vi "灯组解析.vi"() -> ()   [LabVIEW 2015]
uses:
  <userlib>/QMH/Message Queue/Support/Enqueue Message (Single).vi
  Global control/global-1.vi
  <vilib>/Instr/_visa.llb/VISA Configure Serial Port (Instr).vi
  <userlib>/QMH/Message Queue/Support/Enqueue Message (Array).vi
  <userlib>/QMH/Message Queue/Message Queue.lvlib
  <userlib>/QMH/User Event - Stop/User Event - Stop.lvlib
panel:
  in  "HostThread":variant
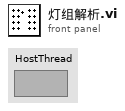
[diagram p1: front panel]
types:
  T1 = cluster{"Controls":cluster{"Exit":refnum<vi>}, "Thread":cluster{"ThisQ":string, "ThisVI":refnum<vi>, "HostQ":string, "HostRef":refnum<vi>, "SlavesQ":string[], "SlavesRef":refnum<vi>[]}, "Data":cluster{"Replace":bool}, "User":cluster{"Name":string}, "长度1-1":cluster{"225":bool, "201":bool, "202":bool, "226":bool, "236":bool, "236-7":bool, "237":bool, "237-7":bool, "231":bool, "231-7":bool, "245":bool, "2451":bool, "241":bool, "241-7":bool, "备用1":bool, "备用2":bool}, "长度2":cluster{"65":bool, "75":bool, "401":bool, "402":bool, "445":bool, "404":bool, "213":bool, "2130":bool, "2131":bool, "405":bool, "406":bool, "407":bool, "备用1":bool, "备用2":bool, "备用3":bool, "备用4":bool}, "长度1-2":cluster{"60":bool, "70":bool, "2120":bool, "212":bool, "2121":bool, "2124":bool, "214":bool, "2140":bool, "2141":bool, "90":bool, "2110":bool, "211":bool, "2111":bool, "2113":bool, "备用1":bool, "备用2":bool}, "VISA":refnum<visa-resource-name>, "1-1":cluster{"225":refnum<vi>, "201":refnum<vi>, "202":refnum<vi>, "226":refnum<vi>, "236":refnum<vi>, "236-7":refnum<vi>, "237":refnum<vi>, "237-7":refnum<vi>, "231":refnum<vi>, "231-7":refnum<vi>, "245":refnum<vi>, "2451":refnum<vi>, "241":refnum<vi>, "241-7":refnum<vi>}, "1-2":cluster{"60":refnum<vi>, "70":refnum<vi>, "2120":refnum<vi>, "212":refnum<vi>, "2121":refnum<vi>, "2124":refnum<vi>, "214":refnum<vi>, "2140":refnum<vi>, "2141":refnum<vi>, "90":refnum<vi>, "2110":refnum<vi>, "211":refnum<vi>, "2111":refnum<vi>, "2113":refnum<vi>}, "2":cluster{"65":refnum<vi>, "75":refnum<vi>, "401":refnum<vi>, "402":refnum<vi>, "445":refnum<vi>, "404":refnum<vi>, "213":refnum<vi>, "2130":refnum<vi>, "2131":refnum<vi>, "405":refnum<vi>, "406":refnum<vi>, "407":refnum<vi>}}
  T2 = cluster{"1-1":cluster{"225":refnum<vi>, "201":refnum<vi>, "202":refnum<vi>, "226":refnum<vi>, "236":refnum<vi>, "236-7":refnum<vi>, "237":refnum<vi>, "237-7":refnum<vi>, "231":refnum<vi>, "231-7":refnum<vi>, "245":refnum<vi>, "2451":refnum<vi>, "241":refnum<vi>, "241-7":refnum<vi>}, "1-2":cluster{"60":refnum<vi>, "70":refnum<vi>, "2120":refnum<vi>, "212":refnum<vi>, "2121":refnum<vi>, "2124":refnum<vi>, "214":refnum<vi>, "2140":refnum<vi>, "2141":refnum<vi>, "90":refnum<vi>, "2110":refnum<vi>, "211":refnum<vi>, "2111":refnum<vi>, "2113":refnum<vi>}, "2":cluster{"65":refnum<vi>, "75":refnum<vi>, "401":refnum<vi>, "402":refnum<vi>, "445":refnum<vi>, "404":refnum<vi>, "213":refnum<vi>, "2130":refnum<vi>, "2131":refnum<vi>, "405":refnum<vi>, "406":refnum<vi>, "407":refnum<vi>}}
  T3 = cluster{"225":bool, "201":bool, "202":bool, "226":bool, "236":bool, "236-7":bool, "237":bool, "237-7":bool, "231":bool, "231-7":bool, "245":bool, "2451":bool, "241":bool, "241-7":bool, "备用1":bool, "备用2":bool}
  T4 = cluster{"225":refnum<vi>, "201":refnum<vi>, "202":refnum<vi>, "226":refnum<vi>, "236":refnum<vi>, "236-7":refnum<vi>, "237":refnum<vi>, "237-7":refnum<vi>, "231":refnum<vi>, "231-7":refnum<vi>, "245":refnum<vi>, "2451":refnum<vi>, "241":refnum<vi>, "241-7":refnum<vi>}
  T5 = cluster{"60":refnum<vi>, "70":refnum<vi>, "2120":refnum<vi>, "212":refnum<vi>, "2121":refnum<vi>, "2124":refnum<vi>, "214":refnum<vi>, "2140":refnum<vi>, "2141":refnum<vi>, "90":refnum<vi>, "2110":refnum<vi>, "211":refnum<vi>, "2111":refnum<vi>, "2113":refnum<vi>}
  T6 = cluster{"65":refnum<vi>, "75":refnum<vi>, "401":refnum<vi>, "402":refnum<vi>, "445":refnum<vi>, "404":refnum<vi>, "213":refnum<vi>, "2130":refnum<vi>, "2131":refnum<vi>, "405":refnum<vi>, "406":refnum<vi>, "407":refnum<vi>}
  T7 = cluster{"60":bool, "70":bool, "2120":bool, "212":bool, "2121":bool, "2124":bool, "214":bool, "2140":bool, "2141":bool, "90":bool, "2110":bool, "211":bool, "2111":bool, "2113":bool, "备用1":bool, "备用2":bool}
  T8 = cluster{"65":bool, "75":bool, "401":bool, "402":bool, "445":bool, "404":bool, "213":bool, "2130":bool, "2131":bool, "405":bool, "406":bool, "407":bool, "备用1":bool, "备用2":bool, "备用3":bool, "备用4":bool}
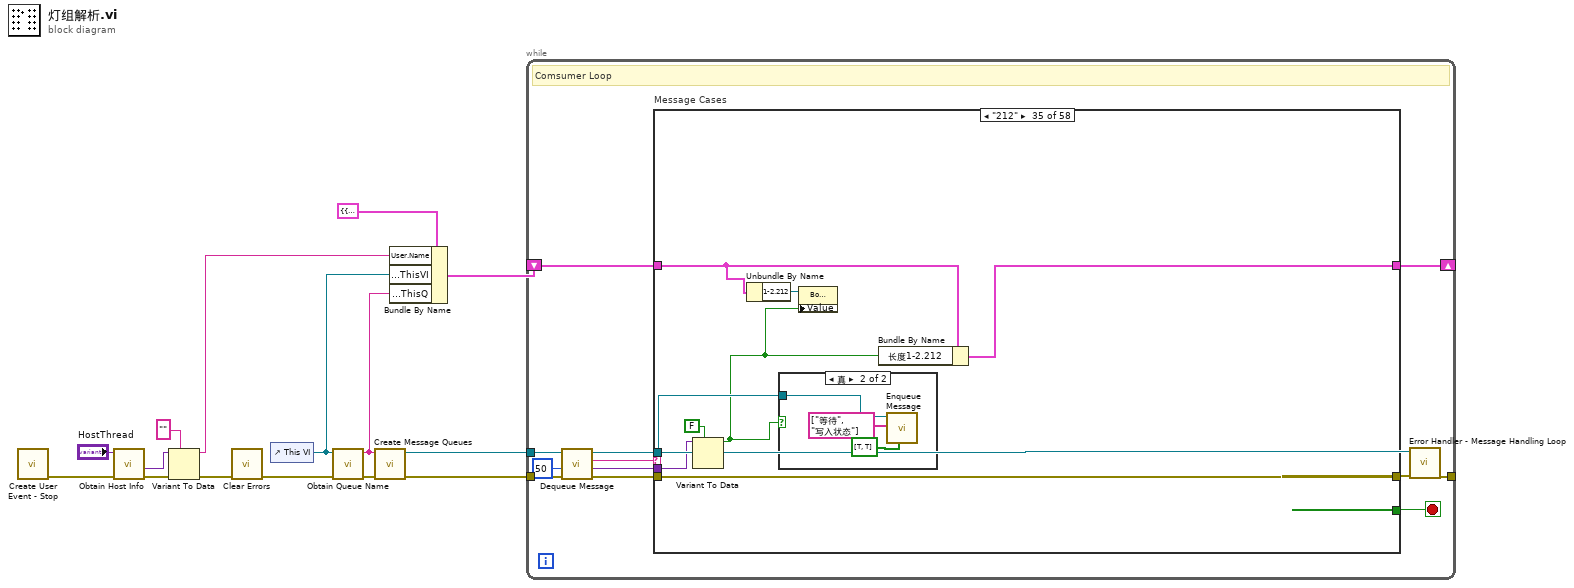
[diagram p0: block diagram]
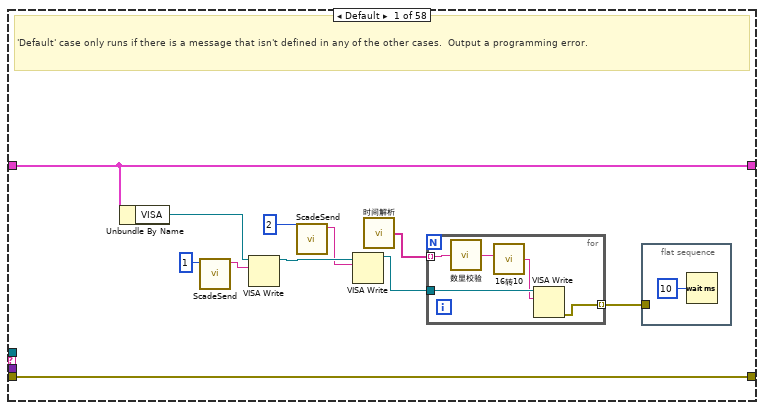
[diagram p2: hidden frame]
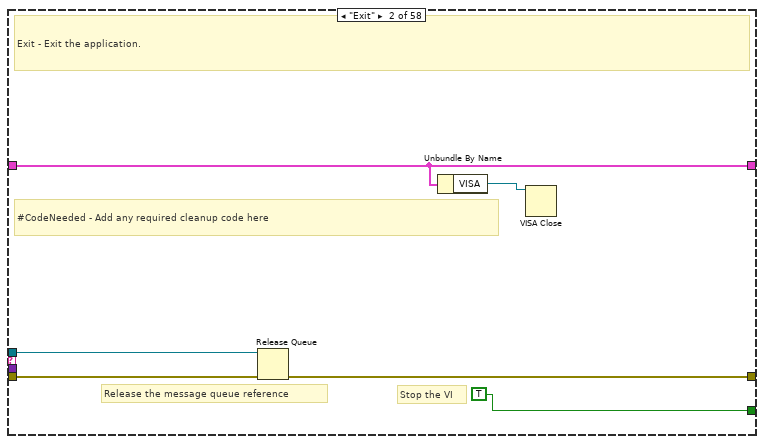
[diagram p3: hidden frame]
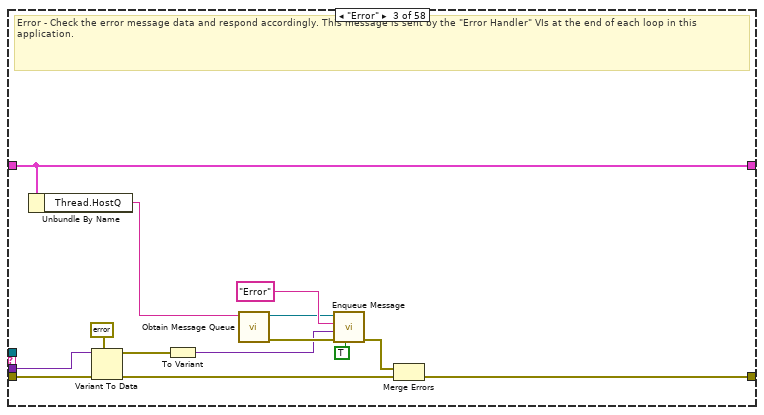
[diagram p4: hidden frame]
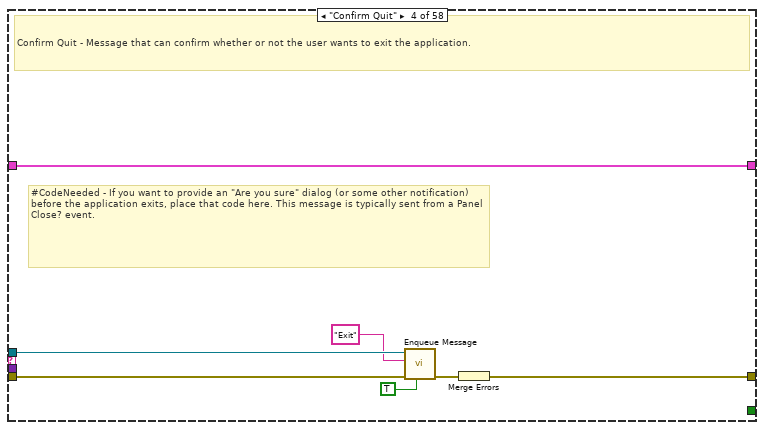
[diagram p5: hidden frame]
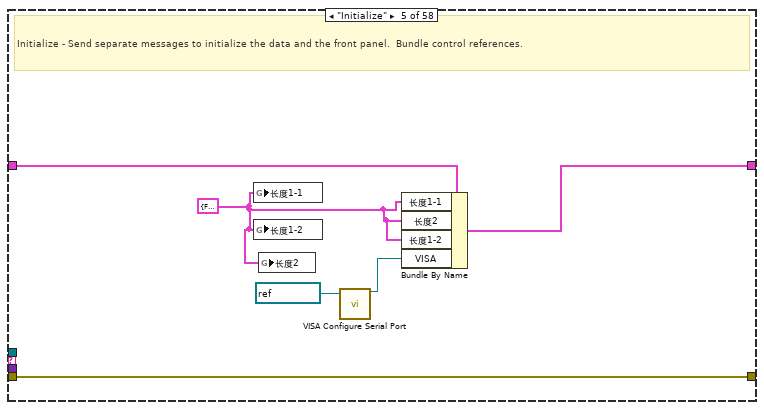
[diagram p6: hidden frame]
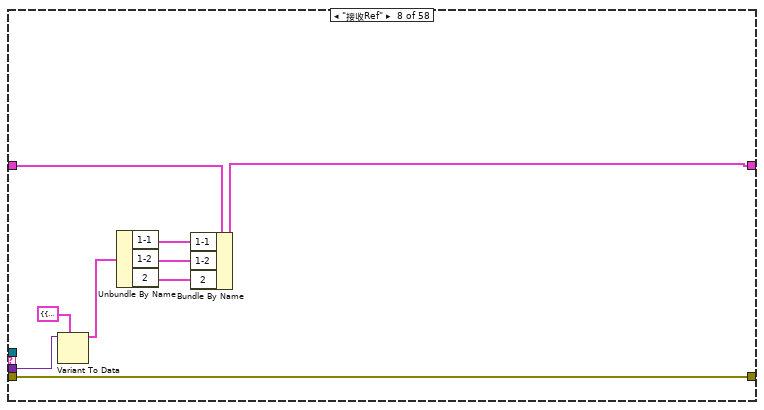
[diagram p9: hidden frame]
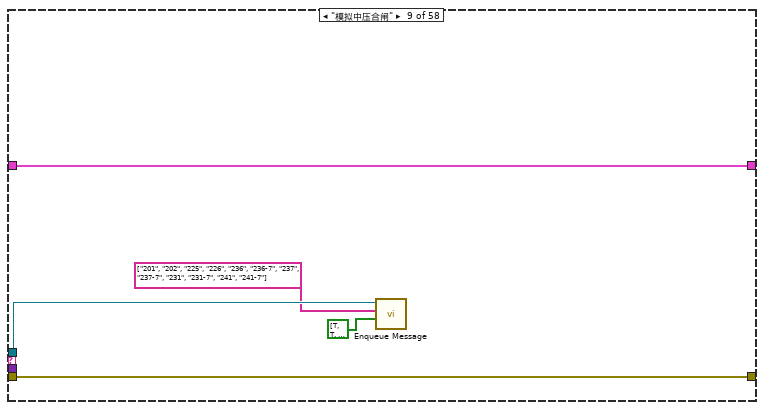
[diagram p10: hidden frame]
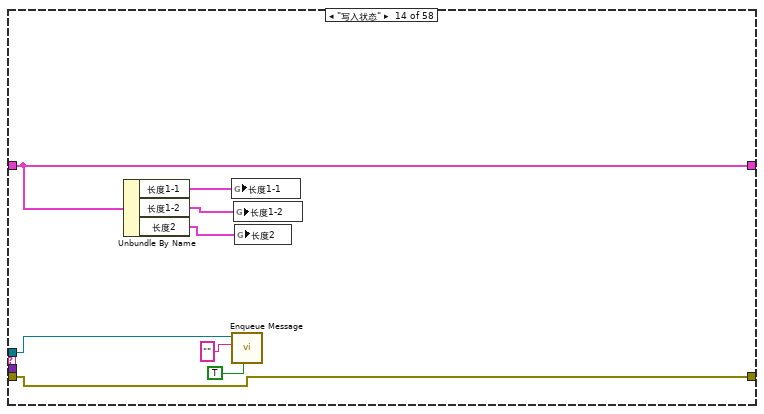
[diagram p15: hidden frame]
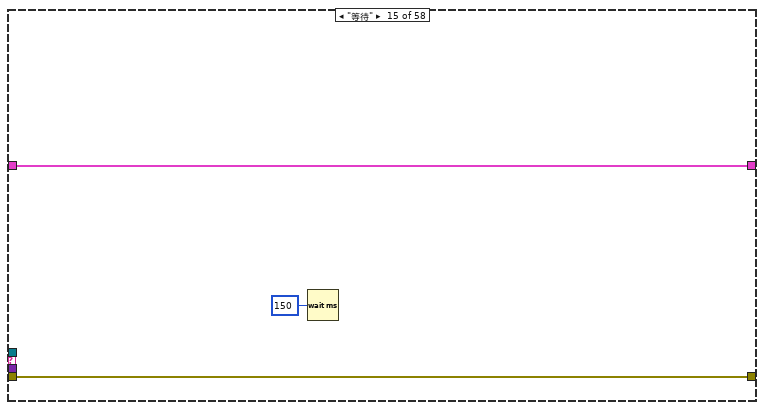
[diagram p16: hidden frame]
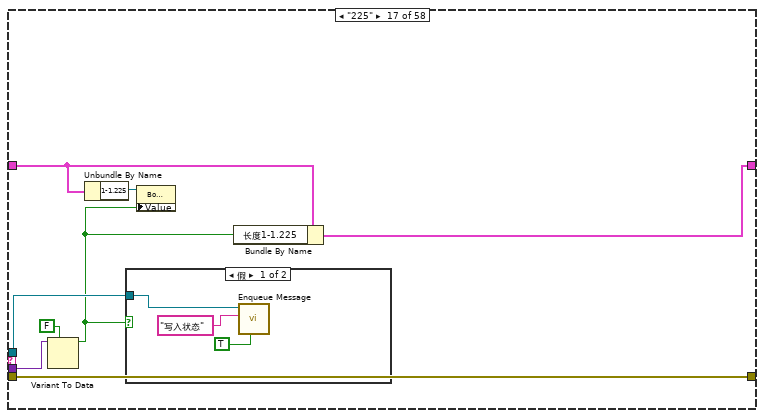
[diagram p18: hidden frame]
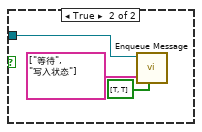
[diagram p19: hidden frame]
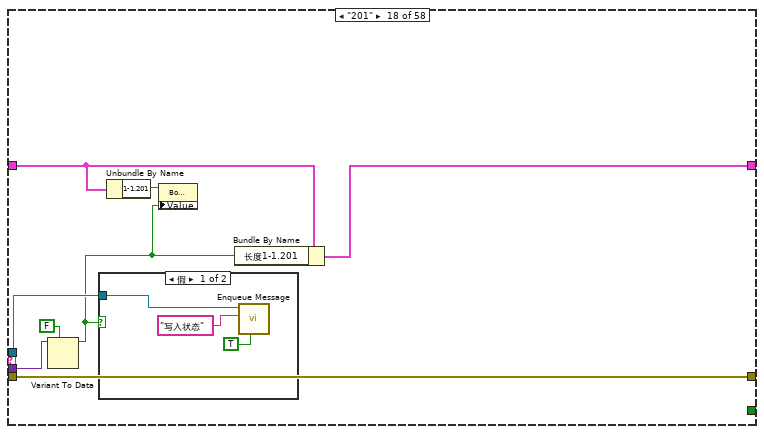
[diagram p20: hidden frame]
diagram:
  n1 = call <userlib>:"Create User Event - Stop.vi"() -> ("error out"=w9:errorcluster)  [unwired: 9 in, 2 out]
  n2 = call <userlib>:"Obtain Host Info.vi"("error in (no error)"=w9, "HostThread"="HostThread") -> ("error out"=w7:errorcluster, "Data"=w6:variant)  [unwired: 6 in, 2 out]
  n3 = Variant To Data(error in=w7, type="", Variant=w6) -> (data=w2:string, error out=w4:errorcluster)
  n4 = call <vilib>:"Clear Errors.vi"("error in (no error)"=w4) -> ("error out"=w3:errorcluster)  [unwired: 5 in, 1 out]
  n5 = control-ref of="This VI"() -> (w11:refnum<vi>)
  n6 = call <userlib>:"Obtain Queue Name.vi"("error in (no error)"=w3, "VI Refnum"=w11) -> ("error out"=w14:errorcluster, "ViName"=w10:string)  [unwired: 8 in]
  n7 = call <userlib>:"Create Message Queues.vi"("error in (no error)"=w14, "name (unnamed)"=w10) -> ("error out"=w15:errorcluster, "QueueHandler"=w1:refnum<queue>)  [unwired: 8 in]
  n8 = Bundle By Name(cluster=T1 {"Controls"={"Exit"=refnum}, "Thread"={"ThisQ"="", "ThisVI"=refnum, "HostQ"="", "HostRef"=refnum, "SlavesQ"=[], "SlavesRef"=[]}, "Data"={"Replace"=FALSE}, "User"={"Name"=""}, "长度1-1"={"225"=FALSE, "201"=FALSE, "202"=FALSE, "226"=FALSE, "236"=FALSE, "236-7"=FALSE, "237"=FALSE, "237-7"=FALSE, "231"=FALSE, "231-7"=FALSE, "245"=FALSE, "2451"=FALSE, "241"=FALSE, "241-7"=FALSE, "备用1"=FALSE, "备用2"=FALSE}, "长度2"={"65"=FALSE, "75"=FALSE, "401"=FALSE, "402"=FALSE, "445"=FALSE, "404"=FALSE, "213"=FALSE, "2130"=FALSE, "2131"=FALSE, "405"=FALSE, "406"=FALSE, "407"=FALSE, "备用1"=FALSE, "备用2"=FALSE, "备用3"=FALSE, "备用4"=FALSE}, "长度1-2"={"60"=FALSE, "70"=FALSE, "2120"=FALSE, "212"=FALSE, "2121"=FALSE, "2124"=FALSE, "214"=FALSE, "2140"=FALSE, "2141"=FALSE, "90"=FALSE, "2110"=FALSE, "211"=FALSE, "2111"=FALSE, "2113"=FALSE, "备用1"=FALSE, "备用2"=FALSE}, "VISA"="", "1-1"={"225"=refnum, "201"=refnum, "202"=refnum, "226"=refnum, "236"=refnum, "236-7"=refnum, "237"=refnum, "237-7"=refnum, "231"=refnum, "231-7"=refnum, "245"=refnum, "2451"=refnum, "241"=refnum, "241-7"=refnum}, "1-2"={"60"=refnum, "70"=refnum, "2120"=refnum, "212"=refnum, "2121"=refnum, "2124"=refnum, "214"=refnum, "2140"=refnum, "2141"=refnum, "90"=refnum, "2110"=refnum, "211"=refnum, "2111"=refnum, "2113"=refnum}, "2"={"65"=refnum, "75"=refnum, "401"=refnum, "402"=refnum, "445"=refnum, "404"=refnum, "213"=refnum, "2130"=refnum, "2131"=refnum, "405"=refnum, "406"=refnum, "407"=refnum}} ("Data Cluster"), "User.Name"=w2, "Thread.ThisVI"=w11, "Thread.ThisQ"=w10) -> (w12:T1)
  n9 = while {
    tunnel: w1 -> [w20]
    shift-right: [w26] -> _
    shift-left: w12 -> [w27]
    tunnel: w15 -> [w24]
    tunnel: [w18] -> _
    stop <- w25 stop-if-true
    # "Comsumer Loop"
    n10 = call <userlib>:"Dequeue Message.vi"("error in (no error)"=w24, "timeout in ms (-1)"=50, "Message Queue"=w20) -> ("error out"=w23:errorcluster, "Message Data"=w21:variant, "Message"=w22:string, "dup Message Queue"=w19:refnum<queue>)  [unwired: 5 in]
    n11 = case "Message Cases" shown="\"212\"" w22 {
      tunnel: w19 -> [_ w50 _ w67 _ _ _ _ w93 _ _ _ _ w106 _ _ w120 w134 w148 w162 w176 w190 w204 w218 w232 w246 w260 w274 w288 w302 _ w318 w332 w346 w360 w374 w388 w402 w416 w430 w444 w458 w472 w486 w500 _ w516 w530 w544 w558 w572 w586 w600 w614 w628 w642 w656 w670]
      tunnel: w23 -> [w30 w48 w64 w71 w77 w79 w81 w90 w95 w97 w98 w101 w103 w111 w114 w116 w124 w138 w152 w166 w180 w194 w208 w222 w236 w250 w264 w278 w292 w306 w314 w322 w336 w350 w364 w378 w392 w406 w420 w434 w448 w462 w476 w490 w504 w512 w520 w534 w548 w562 w576 w590 w604 w618 w632 w646 w660 w674]
      tunnel: [w30 w47 w59 w69 w77 w79 w81 w90 w95 w97 w98 w101 w103 w111 w114 w116 w124 w138 w152 w166 w180 w194 w208 w222 w236 w250 w264 w278 w292 w306 w314 w322 w336 w350 w364 w378 w392 w406 w420 w434 w448 w462 w476 w490 w504 w512 w520 w534 w548 w562 w576 w590 w604 w618 w632 w646 w660 w674] -> w17
      tunnel: w27 -> [w32 w46 w56 w70 w74 w78 w80 w83 w94 w96 w99 w100 w102 w110 w113 w115 w119 w132 w147 w160 w174 w188 w202 w216 w230 w244 w258 w272 w286 w300 w313 w316 w330 w344 w358 w372 w386 w400 w414 w428 w442 w456 w470 w484 w498 w511 w514 w528 w542 w556 w570 w584 w598 w612 w626 w640 w654 w668]
      tunnel: [w32 w46 w56 w70 w73 w78 w80 w82 w94 w96 w99 w100 w102 w110 w113 w115 w121 w135 w149 w163 w177 w191 w205 w219 w233 w247 w261 w275 w289 w303 w313 w319 w333 w347 w361 w375 w389 w403 w417 w431 w445 w459 w473 w487 w501 w511 w517 w531 w545 w559 w573 w587 w601 w615 w629 w643 w657 w671] -> w26
      tunnel: [_ TRUE _ _ _ _ _ _ _ _ _ _ _ _ _ _ _ _ _ _ _ _ _ _ _ _ _ _ _ _ _ _ _ _ _ _ _ _ _ _ _ _ _ _ _ _ _ _ _ _ _ _ _ _ _ _ _ _] -> w25
      tunnel: w21 -> [_ _ w63 _ _ _ _ w89 _ _ _ _ _ _ _ _ w123 w137 w151 w165 w179 w193 w207 w221 w235 w249 w263 w277 w291 w305 _ w321 w335 w349 w363 w377 w391 w405 w419 w433 w447 w461 w475 w489 w503 _ w519 w533 w547 w561 w575 w589 w603 w617 w631 w645 w659 w673]
      frame Default {
        # "'Default' case only runs if there is a message that isn't defined in any of the other cases.  Output a programming error."
        n12 = Unbundle By Name(w32) -> ("VISA"=w31:refnum<visa-resource-name>)
        n13 = call "ScadeSend.vi"("长度"=1) -> ("String"=w36:string)  [unwired: 10 in]
        n14 = VISA Write(VISA resource name=w31, write buffer=w36) -> (VISA resource name out=w35:refnum<visa-resource-name>)  [unwired: 1 in, 2 out]
        n15 = call "ScadeSend.vi"("长度"=2 ("长度 2")) -> ("String"=w34:string)  [unwired: 10 in]
        n16 = VISA Write(VISA resource name=w35, write buffer=w34) -> (VISA resource name out=w37:refnum<visa-resource-name>)  [unwired: 1 in, 2 out]
        n17 = call "时间解析.vi"() -> ("数组"=w33:string[])
        n18 = for {
          tunnel: w33 -> [w41] mode=indexing
          tunnel: w37 -> [w43]
          tunnel: [w40] -> w28 mode=indexing
          n19 = call "数显校验.vi"("字符串"=w41) -> ("连接的字符串"=w44:string)
          n20 = call "16转10.vi"("字符串"=w44) -> ("字符串 2"=w42:string)
          n21 = VISA Write(VISA resource name=w43, write buffer=w42) -> (error out=w40:errorcluster)  [unwired: 1 in, 2 out]
        }
        n22 = flat-sequence {
          tunnel: w28 -> [_]
          frame #0 {
            n23 = Wait (ms)(milliseconds to wait=u32 10 ("等待时间（毫秒）")) -> ()  [unwired: 1 out]
          }
        }
      }
      frame "Exit" {
        # "Stop the VI"
        # "Release the message queue reference"
        # "#CodeNeeded - Add any required cleanup code here"
        # "Exit - Exit the application."
        n24 = Release Queue(queue=w50, error in (no error)=w48) -> (error out=w47:errorcluster)  [unwired: 1 in, 2 out]
        n25 = Unbundle By Name(w46) -> ("VISA"=w45:refnum<visa-resource-name>)
        n26 = VISA Close(VISA resource name=w45) -> ()  [unwired: 1 in, 1 out]
      }
      frame "Error" {
        # "Error - Check the error message data and respond accordingly. This message is sent by the \"Error Handler\" VIs at the end of each loop in this application."
        n27 = Unbundle By Name(w56) -> ("Thread.HostQ"=w55:string)
        n28 = Variant To Data(error in=w64, type=errorcluster {"status"=FALSE, "code"=0, "source"=""} ("error constant"), Variant=w63) -> (data=w52:errorcluster, error out=w61:errorcluster)
        n29 = To Variant(anything=w52) -> (Variant=w51:variant)
        n30 = call <userlib>:"Obtain Message Queue.vi"("name (unnamed)"=w55) -> ("error out"=w54:errorcluster, "Message Queue"=w53:refnum<queue>)  [unwired: 9 in]
        n31 = call-poly <userlib>:"Enqueue Message.vi"("Priority Message? (F)"=TRUE, "error in (no error)"=w54, "Message Data"=w51, "Message"="Error", "Message Queue"=w53) -> ("error out"=w60:errorcluster)  [unwired: 5 in, 1 out]
        n32 = Merge Errors(w60, w61) -> (w59:errorcluster)
      }
      frame "Confirm Quit" {
        # "#CodeNeeded - If you want to provide an \"Are you sure\" dialog (or some other notification) before the application exits, place that code here. This message is typically sent from a Panel Close? event."
        # "Confirm Quit - Message that can confirm whether or not the user wants to exit the application."
        n33 = call-poly <userlib>:"Enqueue Message.vi"("Priority Message? (F)"=TRUE, "error in (no error)"=w71, "Message"="Exit", "Message Queue"=w67) -> ("error out"=w68:errorcluster)  [unwired: 6 in, 1 out]
        n34 = Merge Errors(w68) -> (w69:errorcluster)
      }
      frame "Initialize" {
        w76 = T3 {"225"=FALSE, "201"=FALSE, "202"=FALSE, "226"=FALSE, "236"=FALSE, "236-7"=FALSE, "237"=FALSE, "237-7"=FALSE, "231"=FALSE, "231-7"=FALSE, "245"=FALSE, "2451"=FALSE, "241"=FALSE, "241-7"=FALSE, "备用1"=FALSE, "备用2"=FALSE} ("长度1-1")
        # "Initialize - Send separate messages to initialize the data and the front panel.  Bundle control references."
        n35 = global write "global-1.vi" "长度1-1"(w76) -> ()
        n36 = global write "global-1.vi" "长度1-2"(w76) -> ()
        n37 = global write "global-1.vi" "长度2"(w76) -> ()
        n38 = call-poly "VISA Configure Serial Port"("VISA resource name"=refnum<visa-resource-name> "COM7" ("VISA资源名称")) -> ("VISA resource name out"=w72:refnum<visa-resource-name>)  [unwired: 8 in, 6 out]
        n39 = Bundle By Name(cluster=w74, "长度1-1"=w76, "长度2"=w76, "长度1-2"=w76, "VISA"=w72) -> (w73:T1)
      }
      frame "<-------UI-------->" {
      }
      frame "<------Core------>" {
      }
      frame "接收Ref" {
        n40 = Variant To Data(type=T2 {"1-1"={"225"=refnum, "201"=refnum, "202"=refnum, "226"=refnum, "236"=refnum, "236-7"=refnum, "237"=refnum, "237-7"=refnum, "231"=refnum, "231-7"=refnum, "245"=refnum, "2451"=refnum, "241"=refnum, "241-7"=refnum}, "1-2"={"60"=refnum, "70"=refnum, "2120"=refnum, "212"=refnum, "2121"=refnum, "2124"=refnum, "214"=refnum, "2140"=refnum, "2141"=refnum, "90"=refnum, "2110"=refnum, "211"=refnum, "2111"=refnum, "2113"=refnum}, "2"={"65"=refnum, "75"=refnum, "401"=refnum, "402"=refnum, "445"=refnum, "404"=refnum, "213"=refnum, "2130"=refnum, "2131"=refnum, "405"=refnum, "406"=refnum, "407"=refnum}} ("输出簇"), Variant=w89) -> (data=w87:T2)  [unwired: 1 in, 1 out]
        n41 = Unbundle By Name(w87) -> ("1-1"=w86:T4, "1-2"=w85:T5, "2"=w84:T6)
        n42 = Bundle By Name(cluster=w83, "1-1"=w86, "1-2"=w85, "2"=w84) -> (w82:T1)
      }
      frame "模拟中压合闸" {
        n43 = call-poly <userlib>:"Enqueue Message.vi"("Message Data Array"=bool[] [TRUE, TRUE, TRUE, TRUE, TRUE, TRUE, TRUE, TRUE, TRUE, TRUE, TRUE, TRUE], "Message Array"=string[] ["201", "202", "225", "226", "236", "236-7", "237", "237-7", "231", "231-7", "241", "241-7"], "Message Queue"=w93) -> ()  [unwired: 7 in, 2 out]
      }
      frame "顺序点亮" {
      }
      frame "Core_InitializeRef" {
        # "Initialize control references. For there is not enough space to locate all the control references, separate the codes into 2 messages"
      }
      frame "send" {
      }
      frame "<---Operation--->" {
      }
      frame "写入状态" {
        n44 = Unbundle By Name(w110) -> ("长度1-1"=w109:T3, "长度1-2"=w108:T7, "长度2"=w107:T8)
        n45 = global write "global-1.vi" "长度1-1"(w109) -> ()
        n46 = call-poly <userlib>:"Enqueue Message.vi"("Priority Message? (F)"=TRUE, "Message"="", "Message Queue"=w106) -> ()  [unwired: 7 in, 2 out]
        n47 = global write "global-1.vi" "长度1-2"(w108) -> ()
        n48 = global write "global-1.vi" "长度2"(w107) -> ()
      }
      frame "等待" {
        n49 = Wait (ms)(milliseconds to wait=u32 150 ("等待时间（毫秒）")) -> ()  [unwired: 1 out]
      }
      frame "<-------1-1------->" {
      }
      frame "225" {
        n50 = Variant To Data(type=FALSE, Variant=w123) -> (data=w117:bool)  [unwired: 1 in, 1 out]
        n51 = Unbundle By Name(w119) -> ("1-1.225"=w118:refnum<vi>)
        n52 = case shown="假" w117 {
          tunnel: w120 -> [w127 w130]
          frame False {
            n53 = call-poly <userlib>:"Enqueue Message.vi"("Priority Message? (F)"=TRUE, "Message"="写入状态", "Message Queue"=w127) -> ()  [unwired: 7 in, 2 out]
          }
          frame True {
            n54 = call-poly <userlib>:"Enqueue Message.vi"("Priority Message? Array"=bool[] [TRUE, TRUE], "Message Array"=string[] ["等待", "写入状态"] ("Message"), "Message Queue"=w130) -> ()  [unwired: 7 in, 2 out]
          }
        }
        n55 = property class="Bool (严格)"(reference=w118, "Value"=w117) -> ()  [unwired: 1 in, 2 out]
        n56 = Bundle By Name(cluster=w119, "长度1-1.225"=w117) -> (w121:T1)
      }
      frame "201" {
        n57 = Variant To Data(type=FALSE, Variant=w137) -> (data=w131:bool)  [unwired: 1 in, 1 out]
        n58 = case shown="假" w131 {
          tunnel: w134 -> [w141 w144]
          frame False {
            n59 = call-poly <userlib>:"Enqueue Message.vi"("Priority Message? (F)"=TRUE, "Message"="写入状态", "Message Queue"=w141) -> ()  [unwired: 7 in, 2 out]
          }
          frame True {
            n60 = call-poly <userlib>:"Enqueue Message.vi"("Priority Message? Array"=bool[] [TRUE, TRUE], "Message Array"=string[] ["等待", "写入状态"] ("Message"), "Message Queue"=w144) -> ()  [unwired: 7 in, 2 out]
          }
        }
        n61 = Unbundle By Name(w132) -> ("1-1.201"=w133:refnum<vi>)
        n62 = property class="Bool (严格)"(reference=w133, "Value"=w131) -> ()  [unwired: 1 in, 2 out]
        n63 = Bundle By Name(cluster=w132, "长度1-1.201"=w131) -> (w135:T1)
      }
      frame "202" {
        n64 = Variant To Data(type=FALSE, Variant=w151) -> (data=w145:bool)  [unwired: 1 in, 1 out]
        n65 = Unbundle By Name(w147) -> ("1-1.202"=w146:refnum<vi>)
        n66 = case shown="真" w145 {
          tunnel: w148 -> [w155 w158]
          frame False {
            n67 = call-poly <userlib>:"Enqueue Message.vi"("Priority Message? (F)"=TRUE, "Message"="写入状态", "Message Queue"=w155) -> ()  [unwired: 7 in, 2 out]
          }
          frame True {
            n68 = call-poly <userlib>:"Enqueue Message.vi"("Priority Message? Array"=bool[] [TRUE, TRUE], "Message Array"=string[] ["等待", "写入状态"] ("Message"), "Message Queue"=w158) -> ()  [unwired: 7 in, 2 out]
          }
        }
        n69 = property class="Bool (严格)"(reference=w146, "Value"=w145) -> ()  [unwired: 1 in, 2 out]
        n70 = Bundle By Name(cluster=w147, "长度1-1.202"=w145) -> (w149:T1)
      }
      frame "226" {
        n71 = Variant To Data(type=FALSE, Variant=w165) -> (data=w159:bool)  [unwired: 1 in, 1 out]
        n72 = Unbundle By Name(w160) -> ("1-1.226"=w161:refnum<vi>)
        n73 = case shown="真" w159 {
          tunnel: w162 -> [w169 w172]
          frame False {
            n74 = call-poly <userlib>:"Enqueue Message.vi"("Priority Message? (F)"=TRUE, "Message"="写入状态", "Message Queue"=w169) -> ()  [unwired: 7 in, 2 out]
          }
          frame True {
            n75 = call-poly <userlib>:"Enqueue Message.vi"("Priority Message? Array"=bool[] [TRUE, TRUE], "Message Array"=string[] ["等待", "写入状态"] ("Message"), "Message Queue"=w172) -> ()  [unwired: 7 in, 2 out]
          }
        }
        n76 = property class="Bool (严格)"(reference=w161, "Value"=w159) -> ()  [unwired: 1 in, 2 out]
        n77 = Bundle By Name(cluster=w160, "长度1-1.226"=w159) -> (w163:T1)
      }
      frame "236" {
        n78 = Variant To Data(type=FALSE, Variant=w179) -> (data=w173:bool)  [unwired: 1 in, 1 out]
        n79 = Unbundle By Name(w174) -> ("1-1.236"=w175:refnum<vi>)
        n80 = case shown="真" w173 {
          tunnel: w176 -> [w183 w186]
          frame False {
            n81 = call-poly <userlib>:"Enqueue Message.vi"("Priority Message? (F)"=TRUE, "Message"="写入状态", "Message Queue"=w183) -> ()  [unwired: 7 in, 2 out]
          }
          frame True {
            n82 = call-poly <userlib>:"Enqueue Message.vi"("Priority Message? Array"=bool[] [TRUE, TRUE], "Message Array"=string[] ["等待", "写入状态"] ("Message"), "Message Queue"=w186) -> ()  [unwired: 7 in, 2 out]
          }
        }
        n83 = property class="Bool (严格)"(reference=w175, "Value"=w173) -> ()  [unwired: 1 in, 2 out]
        n84 = Bundle By Name(cluster=w174, "长度1-1.236"=w173) -> (w177:T1)
      }
      frame "236-7" {
        n85 = Variant To Data(type=FALSE, Variant=w193) -> (data=w187:bool)  [unwired: 1 in, 1 out]
        n86 = Unbundle By Name(w188) -> ("1-1.236-7"=w189:refnum<vi>)
        n87 = case shown="真" w187 {
          tunnel: w190 -> [w197 w200]
          frame False {
            n88 = call-poly <userlib>:"Enqueue Message.vi"("Priority Message? (F)"=TRUE, "Message"="写入状态", "Message Queue"=w197) -> ()  [unwired: 7 in, 2 out]
          }
          frame True {
            n89 = call-poly <userlib>:"Enqueue Message.vi"("Priority Message? Array"=bool[] [TRUE, TRUE], "Message Array"=string[] ["等待", "写入状态"] ("Message"), "Message Queue"=w200) -> ()  [unwired: 7 in, 2 out]
          }
        }
        n90 = property class="Bool (严格)"(reference=w189, "Value"=w187) -> ()  [unwired: 1 in, 2 out]
        n91 = Bundle By Name(cluster=w188, "长度1-1.236-7"=w187) -> (w191:T1)
      }
      frame "237" {
        n92 = Variant To Data(type=FALSE, Variant=w207) -> (data=w201:bool)  [unwired: 1 in, 1 out]
        n93 = Unbundle By Name(w202) -> ("1-1.237"=w203:refnum<vi>)
        n94 = case shown="真" w201 {
          tunnel: w204 -> [w211 w214]
          frame False {
            n95 = call-poly <userlib>:"Enqueue Message.vi"("Priority Message? (F)"=TRUE, "Message"="写入状态", "Message Queue"=w211) -> ()  [unwired: 7 in, 2 out]
          }
          frame True {
            n96 = call-poly <userlib>:"Enqueue Message.vi"("Priority Message? Array"=bool[] [TRUE, TRUE], "Message Array"=string[] ["等待", "写入状态"] ("Message"), "Message Queue"=w214) -> ()  [unwired: 7 in, 2 out]
          }
        }
        n97 = property class="Bool (严格)"(reference=w203, "Value"=w201) -> ()  [unwired: 1 in, 2 out]
        n98 = Bundle By Name(cluster=w202, "长度1-1.237"=w201) -> (w205:T1)
      }
      frame "237-7" {
        n99 = Variant To Data(type=FALSE, Variant=w221) -> (data=w215:bool)  [unwired: 1 in, 1 out]
        n100 = Unbundle By Name(w216) -> ("1-1.237-7"=w217:refnum<vi>)
        n101 = case shown="真" w215 {
          tunnel: w218 -> [w225 w228]
          frame False {
            n102 = call-poly <userlib>:"Enqueue Message.vi"("Priority Message? (F)"=TRUE, "Message"="写入状态", "Message Queue"=w225) -> ()  [unwired: 7 in, 2 out]
          }
          frame True {
            n103 = call-poly <userlib>:"Enqueue Message.vi"("Priority Message? Array"=bool[] [TRUE, TRUE], "Message Array"=string[] ["等待", "写入状态"] ("Message"), "Message Queue"=w228) -> ()  [unwired: 7 in, 2 out]
          }
        }
        n104 = property class="Bool (严格)"(reference=w217, "Value"=w215) -> ()  [unwired: 1 in, 2 out]
        n105 = Bundle By Name(cluster=w216, "长度1-1.237-7"=w215) -> (w219:T1)
      }
      frame "231" {
        n106 = Variant To Data(type=FALSE, Variant=w235) -> (data=w229:bool)  [unwired: 1 in, 1 out]
        n107 = Unbundle By Name(w230) -> ("1-1.231"=w231:refnum<vi>)
        n108 = case shown="真" w229 {
          tunnel: w232 -> [w239 w242]
          frame False {
            n109 = call-poly <userlib>:"Enqueue Message.vi"("Priority Message? (F)"=TRUE, "Message"="写入状态", "Message Queue"=w239) -> ()  [unwired: 7 in, 2 out]
          }
          frame True {
            n110 = call-poly <userlib>:"Enqueue Message.vi"("Priority Message? Array"=bool[] [TRUE, TRUE], "Message Array"=string[] ["等待", "写入状态"] ("Message"), "Message Queue"=w242) -> ()  [unwired: 7 in, 2 out]
          }
        }
        n111 = property class="Bool (严格)"(reference=w231, "Value"=w229) -> ()  [unwired: 1 in, 2 out]
        n112 = Bundle By Name(cluster=w230, "长度1-1.231"=w229) -> (w233:T1)
      }
      frame "231-7" {
        n113 = Variant To Data(type=FALSE, Variant=w249) -> (data=w243:bool)  [unwired: 1 in, 1 out]
        n114 = Unbundle By Name(w244) -> ("1-1.231-7"=w245:refnum<vi>)
        n115 = property class="Bool (严格)"(reference=w245, "Value"=w243) -> ()  [unwired: 1 in, 2 out]
        n116 = case shown="真" w243 {
          tunnel: w246 -> [w253 w256]
          frame False {
            n117 = call-poly <userlib>:"Enqueue Message.vi"("Priority Message? (F)"=TRUE, "Message"="写入状态", "Message Queue"=w253) -> ()  [unwired: 7 in, 2 out]
          }
          frame True {
            n118 = call-poly <userlib>:"Enqueue Message.vi"("Priority Message? Array"=bool[] [TRUE, TRUE], "Message Array"=string[] ["等待", "写入状态"] ("Message"), "Message Queue"=w256) -> ()  [unwired: 7 in, 2 out]
          }
        }
        n119 = Bundle By Name(cluster=w244, "长度1-1.231-7"=w243) -> (w247:T1)
      }
      frame "245" {
        n120 = Variant To Data(type=FALSE, Variant=w263) -> (data=w257:bool)  [unwired: 1 in, 1 out]
        n121 = Unbundle By Name(w258) -> ("1-1.245"=w259:refnum<vi>)
        n122 = property class="Bool (严格)"(reference=w259, "Value"=w257) -> ()  [unwired: 1 in, 2 out]
        n123 = case shown="真" w257 {
          tunnel: w260 -> [w267 w270]
          frame False {
            n124 = call-poly <userlib>:"Enqueue Message.vi"("Priority Message? (F)"=TRUE, "Message"="写入状态", "Message Queue"=w267) -> ()  [unwired: 7 in, 2 out]
          }
          frame True {
            n125 = call-poly <userlib>:"Enqueue Message.vi"("Priority Message? Array"=bool[] [TRUE, TRUE], "Message Array"=string[] ["等待", "写入状态"] ("Message"), "Message Queue"=w270) -> ()  [unwired: 7 in, 2 out]
          }
        }
        n126 = Bundle By Name(cluster=w258, "长度1-1.245"=w257) -> (w261:T1)
      }
      frame "2451" {
        n127 = Variant To Data(type=FALSE, Variant=w277) -> (data=w271:bool)  [unwired: 1 in, 1 out]
        n128 = Unbundle By Name(w272) -> ("1-1.2451"=w273:refnum<vi>)
        n129 = case shown="真" w271 {
          tunnel: w274 -> [w281 w284]
          frame False {
            n130 = call-poly <userlib>:"Enqueue Message.vi"("Priority Message? (F)"=TRUE, "Message"="写入状态", "Message Queue"=w281) -> ()  [unwired: 7 in, 2 out]
          }
          frame True {
            n131 = call-poly <userlib>:"Enqueue Message.vi"("Priority Message? Array"=bool[] [TRUE, TRUE], "Message Array"=string[] ["等待", "写入状态"] ("Message"), "Message Queue"=w284) -> ()  [unwired: 7 in, 2 out]
          }
        }
        n132 = property class="Bool (严格)"(reference=w273, "Value"=w271) -> ()  [unwired: 1 in, 2 out]
        n133 = Bundle By Name(cluster=w272, "长度1-1.2451"=w271) -> (w275:T1)
      }
      frame "241" {
        n134 = Variant To Data(type=FALSE, Variant=w291) -> (data=w285:bool)  [unwired: 1 in, 1 out]
        n135 = Unbundle By Name(w286) -> ("1-1.241"=w287:refnum<vi>)
        n136 = case shown="真" w285 {
          tunnel: w288 -> [w295 w298]
          frame False {
            n137 = call-poly <userlib>:"Enqueue Message.vi"("Priority Message? (F)"=TRUE, "Message"="写入状态", "Message Queue"=w295) -> ()  [unwired: 7 in, 2 out]
          }
          frame True {
            n138 = call-poly <userlib>:"Enqueue Message.vi"("Priority Message? Array"=bool[] [TRUE, TRUE], "Message Array"=string[] ["等待", "写入状态"] ("Message"), "Message Queue"=w298) -> ()  [unwired: 7 in, 2 out]
          }
        }
        n139 = property class="Bool (严格)"(reference=w287, "Value"=w285) -> ()  [unwired: 1 in, 2 out]
        n140 = Bundle By Name(cluster=w286, "长度1-1.241"=w285) -> (w289:T1)
      }
      frame "241-7" {
        n141 = Variant To Data(type=FALSE, Variant=w305) -> (data=w299:bool)  [unwired: 1 in, 1 out]
        n142 = Unbundle By Name(w300) -> ("1-1.241-7"=w301:refnum<vi>)
        n143 = case shown="真" w299 {
          tunnel: w302 -> [w309 w312]
          frame False {
            n144 = call-poly <userlib>:"Enqueue Message.vi"("Priority Message? (F)"=TRUE, "Message"="写入状态", "Message Queue"=w309) -> ()  [unwired: 7 in, 2 out]
          }
          frame True {
            n145 = call-poly <userlib>:"Enqueue Message.vi"("Priority Message? Array"=bool[] [TRUE, TRUE], "Message Array"=string[] ["等待", "写入状态"] ("Message"), "Message Queue"=w312) -> ()  [unwired: 7 in, 2 out]
          }
        }
        n146 = property class="Bool (严格)"(reference=w301, "Value"=w299) -> ()  [unwired: 1 in, 2 out]
        n147 = Bundle By Name(cluster=w300, "长度1-1.241-7"=w299) -> (w303:T1)
      }
      frame "<-------1-2------->" {
      }
      frame "60" {
        n148 = Variant To Data(type=FALSE, Variant=w321) -> (data=w315:bool)  [unwired: 1 in, 1 out]
        n149 = Unbundle By Name(w316) -> ("1-2.60"=w317:refnum<vi>)
        n150 = case shown="真" w315 {
          tunnel: w318 -> [w325 w328]
          frame False {
            n151 = call-poly <userlib>:"Enqueue Message.vi"("Priority Message? (F)"=TRUE, "Message"="写入状态", "Message Queue"=w325) -> ()  [unwired: 7 in, 2 out]
          }
          frame True {
            n152 = call-poly <userlib>:"Enqueue Message.vi"("Priority Message? Array"=bool[] [TRUE, TRUE], "Message Array"=string[] ["等待", "写入状态"] ("Message"), "Message Queue"=w328) -> ()  [unwired: 7 in, 2 out]
          }
        }
        n153 = property class="Bool (严格)"(reference=w317, "Value"=w315) -> ()  [unwired: 1 in, 2 out]
        n154 = Bundle By Name(cluster=w316, "长度1-2.60"=w315) -> (w319:T1)
      }
      frame "70" {
        n155 = Variant To Data(type=FALSE, Variant=w335) -> (data=w329:bool)  [unwired: 1 in, 1 out]
        n156 = Unbundle By Name(w330) -> ("1-2.70"=w331:refnum<vi>)
        n157 = property class="Bool (严格)"(reference=w331, "Value"=w329) -> ()  [unwired: 1 in, 2 out]
        n158 = case shown="假" w329 {
          tunnel: w332 -> [w339 w342]
          frame False {
            n159 = call-poly <userlib>:"Enqueue Message.vi"("Priority Message? (F)"=TRUE, "Message"="写入状态", "Message Queue"=w339) -> ()  [unwired: 7 in, 2 out]
          }
          frame True {
            n160 = call-poly <userlib>:"Enqueue Message.vi"("Priority Message? Array"=bool[] [TRUE, TRUE], "Message Array"=string[] ["等待", "写入状态"] ("Message"), "Message Queue"=w342) -> ()  [unwired: 7 in, 2 out]
          }
        }
        n161 = Bundle By Name(cluster=w330, "长度1-2.70"=w329) -> (w333:T1)
      }
      frame "2120" {
        n162 = Variant To Data(type=FALSE, Variant=w349) -> (data=w343:bool)  [unwired: 1 in, 1 out]
        n163 = Unbundle By Name(w344) -> ("1-2.2120"=w345:refnum<vi>)
        n164 = case shown="真" w343 {
          tunnel: w346 -> [w353 w356]
          frame False {
            n165 = call-poly <userlib>:"Enqueue Message.vi"("Priority Message? (F)"=TRUE, "Message"="写入状态", "Message Queue"=w353) -> ()  [unwired: 7 in, 2 out]
          }
          frame True {
            n166 = call-poly <userlib>:"Enqueue Message.vi"("Priority Message? Array"=bool[] [TRUE, TRUE], "Message Array"=string[] ["等待", "写入状态"] ("Message"), "Message Queue"=w356) -> ()  [unwired: 7 in, 2 out]
          }
        }
        n167 = property class="Bool (严格)"(reference=w345, "Value"=w343) -> ()  [unwired: 1 in, 2 out]
        n168 = Bundle By Name(cluster=w344, "长度1-2.2120"=w343) -> (w347:T1)
      }
      frame "212" {
        n169 = Variant To Data(type=FALSE, Variant=w363) -> (data=w357:bool)  [unwired: 1 in, 1 out]
        n170 = Unbundle By Name(w358) -> ("1-2.212"=w359:refnum<vi>)
        n171 = case shown="真" w357 {
          tunnel: w360 -> [w367 w370]
          frame False {
            n172 = call-poly <userlib>:"Enqueue Message.vi"("Priority Message? (F)"=TRUE, "Message"="写入状态", "Message Queue"=w367) -> ()  [unwired: 7 in, 2 out]
          }
          frame True {
            n173 = call-poly <userlib>:"Enqueue Message.vi"("Priority Message? Array"=bool[] [TRUE, TRUE], "Message Array"=string[] ["等待", "写入状态"] ("Message"), "Message Queue"=w370) -> ()  [unwired: 7 in, 2 out]
          }
        }
        n174 = property class="Bool (严格)"(reference=w359, "Value"=w357) -> ()  [unwired: 1 in, 2 out]
        n175 = Bundle By Name(cluster=w358, "长度1-2.212"=w357) -> (w361:T1)
      }
      frame "2121" {
        n176 = Variant To Data(type=FALSE, Variant=w377) -> (data=w371:bool)  [unwired: 1 in, 1 out]
        n177 = Unbundle By Name(w372) -> ("1-2.2121"=w373:refnum<vi>)
        n178 = case shown="真" w371 {
          tunnel: w374 -> [w381 w384]
          frame False {
            n179 = call-poly <userlib>:"Enqueue Message.vi"("Priority Message? (F)"=TRUE, "Message"="写入状态", "Message Queue"=w381) -> ()  [unwired: 7 in, 2 out]
          }
          frame True {
            n180 = call-poly <userlib>:"Enqueue Message.vi"("Priority Message? Array"=bool[] [TRUE, TRUE], "Message Array"=string[] ["等待", "写入状态"] ("Message"), "Message Queue"=w384) -> ()  [unwired: 7 in, 2 out]
          }
        }
        n181 = property class="Bool (严格)"(reference=w373, "Value"=w371) -> ()  [unwired: 1 in, 2 out]
        n182 = Bundle By Name(cluster=w372, "长度1-2.2121"=w371) -> (w375:T1)
      }
      frame "2124" {
        n183 = Variant To Data(type=FALSE, Variant=w391) -> (data=w385:bool)  [unwired: 1 in, 1 out]
        n184 = Unbundle By Name(w386) -> ("1-2.2124"=w387:refnum<vi>)
        n185 = case shown="真" w385 {
          tunnel: w388 -> [w395 w398]
          frame False {
            n186 = call-poly <userlib>:"Enqueue Message.vi"("Priority Message? (F)"=TRUE, "Message"="写入状态", "Message Queue"=w395) -> ()  [unwired: 7 in, 2 out]
          }
          frame True {
            n187 = call-poly <userlib>:"Enqueue Message.vi"("Priority Message? Array"=bool[] [TRUE, TRUE], "Message Array"=string[] ["等待", "写入状态"] ("Message"), "Message Queue"=w398) -> ()  [unwired: 7 in, 2 out]
          }
        }
        n188 = property class="Bool (严格)"(reference=w387, "Value"=w385) -> ()  [unwired: 1 in, 2 out]
        n189 = Bundle By Name(cluster=w386, "长度1-2.2124"=w385) -> (w389:T1)
      }
      frame "214" {
        n190 = Variant To Data(type=FALSE, Variant=w405) -> (data=w399:bool)  [unwired: 1 in, 1 out]
        n191 = Unbundle By Name(w400) -> ("1-2.214"=w401:refnum<vi>)
        n192 = case shown="真" w399 {
          tunnel: w402 -> [w409 w412]
          frame False {
            n193 = call-poly <userlib>:"Enqueue Message.vi"("Priority Message? (F)"=TRUE, "Message"="写入状态", "Message Queue"=w409) -> ()  [unwired: 7 in, 2 out]
          }
          frame True {
            n194 = call-poly <userlib>:"Enqueue Message.vi"("Priority Message? Array"=bool[] [TRUE, TRUE], "Message Array"=string[] ["等待", "写入状态"] ("Message"), "Message Queue"=w412) -> ()  [unwired: 7 in, 2 out]
          }
        }
        n195 = property class="Bool (严格)"(reference=w401, "Value"=w399) -> ()  [unwired: 1 in, 2 out]
        n196 = Bundle By Name(cluster=w400, "长度1-2.214"=w399) -> (w403:T1)
      }
      frame "2140" {
        n197 = Variant To Data(type=FALSE, Variant=w419) -> (data=w413:bool)  [unwired: 1 in, 1 out]
        n198 = Unbundle By Name(w414) -> ("1-2.2140"=w415:refnum<vi>)
        n199 = case shown="真" w413 {
          tunnel: w416 -> [w423 w426]
          frame False {
            n200 = call-poly <userlib>:"Enqueue Message.vi"("Priority Message? (F)"=TRUE, "Message"="写入状态", "Message Queue"=w423) -> ()  [unwired: 7 in, 2 out]
          }
          frame True {
            n201 = call-poly <userlib>:"Enqueue Message.vi"("Priority Message? Array"=bool[] [TRUE, TRUE], "Message Array"=string[] ["等待", "写入状态"] ("Message"), "Message Queue"=w426) -> ()  [unwired: 7 in, 2 out]
          }
        }
        n202 = property class="Bool (严格)"(reference=w415, "Value"=w413) -> ()  [unwired: 1 in, 2 out]
        n203 = Bundle By Name(cluster=w414, "长度1-2.2140"=w413) -> (w417:T1)
      }
      frame "2141" {
        n204 = Variant To Data(type=FALSE, Variant=w433) -> (data=w427:bool)  [unwired: 1 in, 1 out]
        n205 = Unbundle By Name(w428) -> ("1-2.2141"=w429:refnum<vi>)
        n206 = case shown="真" w427 {
          tunnel: w430 -> [w437 w440]
          frame False {
            n207 = call-poly <userlib>:"Enqueue Message.vi"("Priority Message? (F)"=TRUE, "Message"="写入状态", "Message Queue"=w437) -> ()  [unwired: 7 in, 2 out]
          }
          frame True {
            n208 = call-poly <userlib>:"Enqueue Message.vi"("Priority Message? Array"=bool[] [TRUE, TRUE], "Message Array"=string[] ["等待", "写入状态"] ("Message"), "Message Queue"=w440) -> ()  [unwired: 7 in, 2 out]
          }
        }
        n209 = property class="Bool (严格)"(reference=w429, "Value"=w427) -> ()  [unwired: 1 in, 2 out]
        n210 = Bundle By Name(cluster=w428, "长度1-2.2141"=w427) -> (w431:T1)
      }
      frame "90" {
        n211 = Variant To Data(type=FALSE, Variant=w447) -> (data=w441:bool)  [unwired: 1 in, 1 out]
        n212 = Unbundle By Name(w442) -> ("1-2.90"=w443:refnum<vi>)
        n213 = case shown="真" w441 {
          tunnel: w444 -> [w451 w454]
          frame False {
            n214 = call-poly <userlib>:"Enqueue Message.vi"("Priority Message? (F)"=TRUE, "Message"="写入状态", "Message Queue"=w451) -> ()  [unwired: 7 in, 2 out]
          }
          frame True {
            n215 = call-poly <userlib>:"Enqueue Message.vi"("Priority Message? Array"=bool[] [TRUE, TRUE], "Message Array"=string[] ["等待", "写入状态"] ("Message"), "Message Queue"=w454) -> ()  [unwired: 7 in, 2 out]
          }
        }
        n216 = property class="Bool (严格)"(reference=w443, "Value"=w441) -> ()  [unwired: 1 in, 2 out]
        n217 = Bundle By Name(cluster=w442, "长度1-2.90"=w441) -> (w445:T1)
      }
      frame "2110" {
        n218 = Variant To Data(type=FALSE, Variant=w461) -> (data=w455:bool)  [unwired: 1 in, 1 out]
        n219 = Unbundle By Name(w456) -> ("1-2.2110"=w457:refnum<vi>)
        n220 = case shown="真" w455 {
          tunnel: w458 -> [w465 w468]
          frame False {
            n221 = call-poly <userlib>:"Enqueue Message.vi"("Priority Message? (F)"=TRUE, "Message"="写入状态", "Message Queue"=w465) -> ()  [unwired: 7 in, 2 out]
          }
          frame True {
            n222 = call-poly <userlib>:"Enqueue Message.vi"("Priority Message? Array"=bool[] [TRUE, TRUE], "Message Array"=string[] ["等待", "写入状态"] ("Message"), "Message Queue"=w468) -> ()  [unwired: 7 in, 2 out]
          }
        }
        n223 = property class="Bool (严格)"(reference=w457, "Value"=w455) -> ()  [unwired: 1 in, 2 out]
        n224 = Bundle By Name(cluster=w456, "长度1-2.2110"=w455) -> (w459:T1)
      }
      frame "211" {
        n225 = Variant To Data(type=FALSE, Variant=w475) -> (data=w469:bool)  [unwired: 1 in, 1 out]
        n226 = Unbundle By Name(w470) -> ("1-2.211"=w471:refnum<vi>)
        n227 = case shown="真" w469 {
          tunnel: w472 -> [w479 w482]
          frame False {
            n228 = call-poly <userlib>:"Enqueue Message.vi"("Priority Message? (F)"=TRUE, "Message"="写入状态", "Message Queue"=w479) -> ()  [unwired: 7 in, 2 out]
          }
          frame True {
            n229 = call-poly <userlib>:"Enqueue Message.vi"("Priority Message? Array"=bool[] [TRUE, TRUE], "Message Array"=string[] ["等待", "写入状态"] ("Message"), "Message Queue"=w482) -> ()  [unwired: 7 in, 2 out]
          }
        }
        n230 = property class="Bool (严格)"(reference=w471, "Value"=w469) -> ()  [unwired: 1 in, 2 out]
        n231 = Bundle By Name(cluster=w470, "长度1-2.211"=w469) -> (w473:T1)
      }
      frame "2111" {
        n232 = Variant To Data(type=FALSE, Variant=w489) -> (data=w483:bool)  [unwired: 1 in, 1 out]
        n233 = Unbundle By Name(w484) -> ("1-2.2111"=w485:refnum<vi>)
        n234 = case shown="真" w483 {
          tunnel: w486 -> [w493 w496]
          frame False {
            n235 = call-poly <userlib>:"Enqueue Message.vi"("Priority Message? (F)"=TRUE, "Message"="写入状态", "Message Queue"=w493) -> ()  [unwired: 7 in, 2 out]
          }
          frame True {
            n236 = call-poly <userlib>:"Enqueue Message.vi"("Priority Message? Array"=bool[] [TRUE, TRUE], "Message Array"=string[] ["等待", "写入状态"] ("Message"), "Message Queue"=w496) -> ()  [unwired: 7 in, 2 out]
          }
        }
        n237 = property class="Bool (严格)"(reference=w485, "Value"=w483) -> ()  [unwired: 1 in, 2 out]
        n238 = Bundle By Name(cluster=w484, "长度1-2.2111"=w483) -> (w487:T1)
      }
      frame "2113" {
        n239 = Variant To Data(type=FALSE, Variant=w503) -> (data=w497:bool)  [unwired: 1 in, 1 out]
        n240 = Unbundle By Name(w498) -> ("1-2.2113"=w499:refnum<vi>)
        n241 = case shown="真" w497 {
          tunnel: w500 -> [w507 w510]
          frame False {
            n242 = call-poly <userlib>:"Enqueue Message.vi"("Priority Message? (F)"=TRUE, "Message"="写入状态", "Message Queue"=w507) -> ()  [unwired: 7 in, 2 out]
          }
          frame True {
            n243 = call-poly <userlib>:"Enqueue Message.vi"("Priority Message? Array"=bool[] [TRUE, TRUE], "Message Array"=string[] ["等待", "写入状态"] ("Message"), "Message Queue"=w510) -> ()  [unwired: 7 in, 2 out]
          }
        }
        n244 = property class="Bool (严格)"(reference=w499, "Value"=w497) -> ()  [unwired: 1 in, 2 out]
        n245 = Bundle By Name(cluster=w498, "长度1-2.2113"=w497) -> (w501:T1)
      }
      frame "<--------2-------->" {
      }
      frame "65" {
        n246 = Variant To Data(type=FALSE, Variant=w519) -> (data=w513:bool)  [unwired: 1 in, 1 out]
        n247 = Unbundle By Name(w514) -> ("2.65"=w515:refnum<vi>)
        n248 = property class="Bool (严格)"(reference=w515, "Value"=w513) -> ()  [unwired: 1 in, 2 out]
        n249 = case shown="真" w513 {
          tunnel: w516 -> [w523 w526]
          frame False {
            n250 = call-poly <userlib>:"Enqueue Message.vi"("Priority Message? (F)"=TRUE, "Message"="写入状态", "Message Queue"=w523) -> ()  [unwired: 7 in, 2 out]
          }
          frame True {
            n251 = call-poly <userlib>:"Enqueue Message.vi"("Priority Message? Array"=bool[] [TRUE, TRUE], "Message Array"=string[] ["等待", "写入状态"] ("Message"), "Message Queue"=w526) -> ()  [unwired: 7 in, 2 out]
          }
        }
        n252 = Bundle By Name(cluster=w514, "长度2.65"=w513) -> (w517:T1)
      }
      frame "75" {
        n253 = Variant To Data(type=FALSE, Variant=w533) -> (data=w527:bool)  [unwired: 1 in, 1 out]
        n254 = Unbundle By Name(w528) -> ("2.75"=w529:refnum<vi>)
        n255 = case shown="真" w527 {
          tunnel: w530 -> [w537 w540]
          frame False {
            n256 = call-poly <userlib>:"Enqueue Message.vi"("Priority Message? (F)"=TRUE, "Message"="写入状态", "Message Queue"=w537) -> ()  [unwired: 7 in, 2 out]
          }
          frame True {
            n257 = call-poly <userlib>:"Enqueue Message.vi"("Priority Message? Array"=bool[] [TRUE, TRUE], "Message Array"=string[] ["等待", "写入状态"] ("Message"), "Message Queue"=w540) -> ()  [unwired: 7 in, 2 out]
          }
        }
        n258 = property class="Bool (严格)"(reference=w529, "Value"=w527) -> ()  [unwired: 1 in, 2 out]
        n259 = Bundle By Name(cluster=w528, "长度2.75"=w527) -> (w531:T1)
      }
      frame "401" {
        n260 = Variant To Data(type=FALSE, Variant=w547) -> (data=w541:bool)  [unwired: 1 in, 1 out]
        n261 = Unbundle By Name(w542) -> ("2.401"=w543:refnum<vi>)
        n262 = case shown="真" w541 {
          tunnel: w544 -> [w551 w554]
          frame False {
            n263 = call-poly <userlib>:"Enqueue Message.vi"("Priority Message? (F)"=TRUE, "Message"="写入状态", "Message Queue"=w551) -> ()  [unwired: 7 in, 2 out]
          }
          frame True {
            n264 = call-poly <userlib>:"Enqueue Message.vi"("Priority Message? Array"=bool[] [TRUE, TRUE], "Message Array"=string[] ["等待", "写入状态"] ("Message"), "Message Queue"=w554) -> ()  [unwired: 7 in, 2 out]
          }
        }
        n265 = property class="Bool (严格)"(reference=w543, "Value"=w541) -> ()  [unwired: 1 in, 2 out]
        n266 = Bundle By Name(cluster=w542, "长度2.401"=w541) -> (w545:T1)
      }
      frame "402" {
        n267 = Variant To Data(type=FALSE, Variant=w561) -> (data=w555:bool)  [unwired: 1 in, 1 out]
        n268 = Unbundle By Name(w556) -> ("2.402"=w557:refnum<vi>)
        n269 = case shown="真" w555 {
          tunnel: w558 -> [w565 w568]
          frame False {
            n270 = call-poly <userlib>:"Enqueue Message.vi"("Priority Message? (F)"=TRUE, "Message"="写入状态", "Message Queue"=w565) -> ()  [unwired: 7 in, 2 out]
          }
          frame True {
            n271 = call-poly <userlib>:"Enqueue Message.vi"("Priority Message? Array"=bool[] [TRUE, TRUE], "Message Array"=string[] ["等待", "写入状态"] ("Message"), "Message Queue"=w568) -> ()  [unwired: 7 in, 2 out]
          }
        }
        n272 = property class="Bool (严格)"(reference=w557, "Value"=w555) -> ()  [unwired: 1 in, 2 out]
        n273 = Bundle By Name(cluster=w556, "长度2.402"=w555) -> (w559:T1)
      }
      frame "445" {
        n274 = Variant To Data(type=FALSE, Variant=w575) -> (data=w569:bool)  [unwired: 1 in, 1 out]
        n275 = Unbundle By Name(w570) -> ("2.445"=w571:refnum<vi>)
        n276 = case shown="真" w569 {
          tunnel: w572 -> [w579 w582]
          frame False {
            n277 = call-poly <userlib>:"Enqueue Message.vi"("Priority Message? (F)"=TRUE, "Message"="写入状态", "Message Queue"=w579) -> ()  [unwired: 7 in, 2 out]
          }
          frame True {
            n278 = call-poly <userlib>:"Enqueue Message.vi"("Priority Message? Array"=bool[] [TRUE, TRUE], "Message Array"=string[] ["等待", "写入状态"] ("Message"), "Message Queue"=w582) -> ()  [unwired: 7 in, 2 out]
          }
        }
        n279 = property class="Bool (严格)"(reference=w571, "Value"=w569) -> ()  [unwired: 1 in, 2 out]
        n280 = Bundle By Name(cluster=w570, "长度2.445"=w569) -> (w573:T1)
      }
      frame "404" {
        n281 = Variant To Data(type=FALSE, Variant=w589) -> (data=w583:bool)  [unwired: 1 in, 1 out]
        n282 = Unbundle By Name(w584) -> ("2.404"=w585:refnum<vi>)
        n283 = case shown="真" w583 {
          tunnel: w586 -> [w593 w596]
          frame False {
            n284 = call-poly <userlib>:"Enqueue Message.vi"("Priority Message? (F)"=TRUE, "Message"="写入状态", "Message Queue"=w593) -> ()  [unwired: 7 in, 2 out]
          }
          frame True {
            n285 = call-poly <userlib>:"Enqueue Message.vi"("Priority Message? Array"=bool[] [TRUE, TRUE], "Message Array"=string[] ["等待", "写入状态"] ("Message"), "Message Queue"=w596) -> ()  [unwired: 7 in, 2 out]
          }
        }
        n286 = property class="Bool (严格)"(reference=w585, "Value"=w583) -> ()  [unwired: 1 in, 2 out]
        n287 = Bundle By Name(cluster=w584, "长度2.404"=w583) -> (w587:T1)
      }
      frame "213" {
        n288 = Variant To Data(type=FALSE, Variant=w603) -> (data=w597:bool)  [unwired: 1 in, 1 out]
        n289 = Unbundle By Name(w598) -> ("2.213"=w599:refnum<vi>)
        n290 = case shown="真" w597 {
          tunnel: w600 -> [w607 w610]
          frame False {
            n291 = call-poly <userlib>:"Enqueue Message.vi"("Priority Message? (F)"=TRUE, "Message"="写入状态", "Message Queue"=w607) -> ()  [unwired: 7 in, 2 out]
          }
          frame True {
            n292 = call-poly <userlib>:"Enqueue Message.vi"("Priority Message? Array"=bool[] [TRUE, TRUE], "Message Array"=string[] ["等待", "写入状态"] ("Message"), "Message Queue"=w610) -> ()  [unwired: 7 in, 2 out]
          }
        }
        n293 = property class="Bool (严格)"(reference=w599, "Value"=w597) -> ()  [unwired: 1 in, 2 out]
        n294 = Bundle By Name(cluster=w598, "长度2.213"=w597) -> (w601:T1)
      }
      frame "2130" {
        n295 = Variant To Data(type=FALSE, Variant=w617) -> (data=w611:bool)  [unwired: 1 in, 1 out]
        n296 = Unbundle By Name(w612) -> ("2.2130"=w613:refnum<vi>)
        n297 = case shown="真" w611 {
          tunnel: w614 -> [w621 w624]
          frame False {
            n298 = call-poly <userlib>:"Enqueue Message.vi"("Priority Message? (F)"=TRUE, "Message"="写入状态", "Message Queue"=w621) -> ()  [unwired: 7 in, 2 out]
          }
          frame True {
            n299 = call-poly <userlib>:"Enqueue Message.vi"("Priority Message? Array"=bool[] [TRUE, TRUE], "Message Array"=string[] ["等待", "写入状态"] ("Message"), "Message Queue"=w624) -> ()  [unwired: 7 in, 2 out]
          }
        }
        n300 = property class="Bool (严格)"(reference=w613, "Value"=w611) -> ()  [unwired: 1 in, 2 out]
        n301 = Bundle By Name(cluster=w612, "长度2.2130"=w611) -> (w615:T1)
      }
      frame "2131" {
        n302 = Variant To Data(type=FALSE, Variant=w631) -> (data=w625:bool)  [unwired: 1 in, 1 out]
        n303 = Unbundle By Name(w626) -> ("2.2131"=w627:refnum<vi>)
        n304 = case shown="真" w625 {
          tunnel: w628 -> [w635 w638]
          frame False {
            n305 = call-poly <userlib>:"Enqueue Message.vi"("Priority Message? (F)"=TRUE, "Message"="写入状态", "Message Queue"=w635) -> ()  [unwired: 7 in, 2 out]
          }
          frame True {
            n306 = call-poly <userlib>:"Enqueue Message.vi"("Priority Message? Array"=bool[] [TRUE, TRUE], "Message Array"=string[] ["等待", "写入状态"] ("Message"), "Message Queue"=w638) -> ()  [unwired: 7 in, 2 out]
          }
        }
        n307 = property class="Bool (严格)"(reference=w627, "Value"=w625) -> ()  [unwired: 1 in, 2 out]
        n308 = Bundle By Name(cluster=w626, "长度2.2131"=w625) -> (w629:T1)
      }
      frame "405" {
        n309 = Variant To Data(type=FALSE, Variant=w645) -> (data=w639:bool)  [unwired: 1 in, 1 out]
        n310 = Unbundle By Name(w640) -> ("2.405"=w641:refnum<vi>)
        n311 = case shown="真" w639 {
          tunnel: w642 -> [w649 w652]
          frame False {
            n312 = call-poly <userlib>:"Enqueue Message.vi"("Priority Message? (F)"=TRUE, "Message"="写入状态", "Message Queue"=w649) -> ()  [unwired: 7 in, 2 out]
          }
          frame True {
            n313 = call-poly <userlib>:"Enqueue Message.vi"("Priority Message? Array"=bool[] [TRUE, TRUE], "Message Array"=string[] ["等待", "写入状态"] ("Message"), "Message Queue"=w652) -> ()  [unwired: 7 in, 2 out]
          }
        }
        n314 = property class="Bool (严格)"(reference=w641, "Value"=w639) -> ()  [unwired: 1 in, 2 out]
        n315 = Bundle By Name(cluster=w640, "长度2.405"=w639) -> (w643:T1)
      }
      frame "406" {
        n316 = Variant To Data(type=FALSE, Variant=w659) -> (data=w653:bool)  [unwired: 1 in, 1 out]
        n317 = Unbundle By Name(w654) -> ("2.406"=w655:refnum<vi>)
        n318 = case shown="真" w653 {
          tunnel: w656 -> [w663 w666]
          frame False {
            n319 = call-poly <userlib>:"Enqueue Message.vi"("Priority Message? (F)"=TRUE, "Message"="写入状态", "Message Queue"=w663) -> ()  [unwired: 7 in, 2 out]
          }
          frame True {
            n320 = call-poly <userlib>:"Enqueue Message.vi"("Priority Message? Array"=bool[] [TRUE, TRUE], "Message Array"=string[] ["等待", "写入状态"] ("Message"), "Message Queue"=w666) -> ()  [unwired: 7 in, 2 out]
          }
        }
        n321 = property class="Bool (严格)"(reference=w655, "Value"=w653) -> ()  [unwired: 1 in, 2 out]
        n322 = Bundle By Name(cluster=w654, "长度2.406"=w653) -> (w657:T1)
      }
      frame "407" {
        n323 = Variant To Data(type=FALSE, Variant=w673) -> (data=w667:bool)  [unwired: 1 in, 1 out]
        n324 = Unbundle By Name(w668) -> ("2.407"=w669:refnum<vi>)
        n325 = case shown="真" w667 {
          tunnel: w670 -> [w677 w680]
          frame False {
            n326 = call-poly <userlib>:"Enqueue Message.vi"("Priority Message? (F)"=TRUE, "Message"="写入状态", "Message Queue"=w677) -> ()  [unwired: 7 in, 2 out]
          }
          frame True {
            n327 = call-poly <userlib>:"Enqueue Message.vi"("Priority Message? Array"=bool[] [TRUE, TRUE], "Message Array"=string[] ["等待", "写入状态"] ("Message"), "Message Queue"=w680) -> ()  [unwired: 7 in, 2 out]
          }
        }
        n328 = property class="Bool (严格)"(reference=w669, "Value"=w667) -> ()  [unwired: 1 in, 2 out]
        n329 = Bundle By Name(cluster=w668, "长度2.407"=w667) -> (w671:T1)
      }
    }
    n330 = call <userlib>:"Error Handler - Message Handling Loop.vi"("error in (no error)"=w17, "Message Queue"=w19) -> ("dup error in"=w18:errorcluster)  [unwired: 8 in, 1 out]
  }
